vi "Host_9.vi"() -> ()   [LabVIEW 2020]
panel:
  in  "stop":bool
  out "Dane":waveform(dbl)(graph)
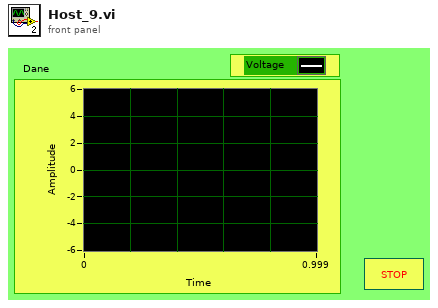
[diagram p1: front panel]
types:
  T1 = enum16{"open", "replace", "create", "open or create", "replace or create", "replace or create with confirmation"}
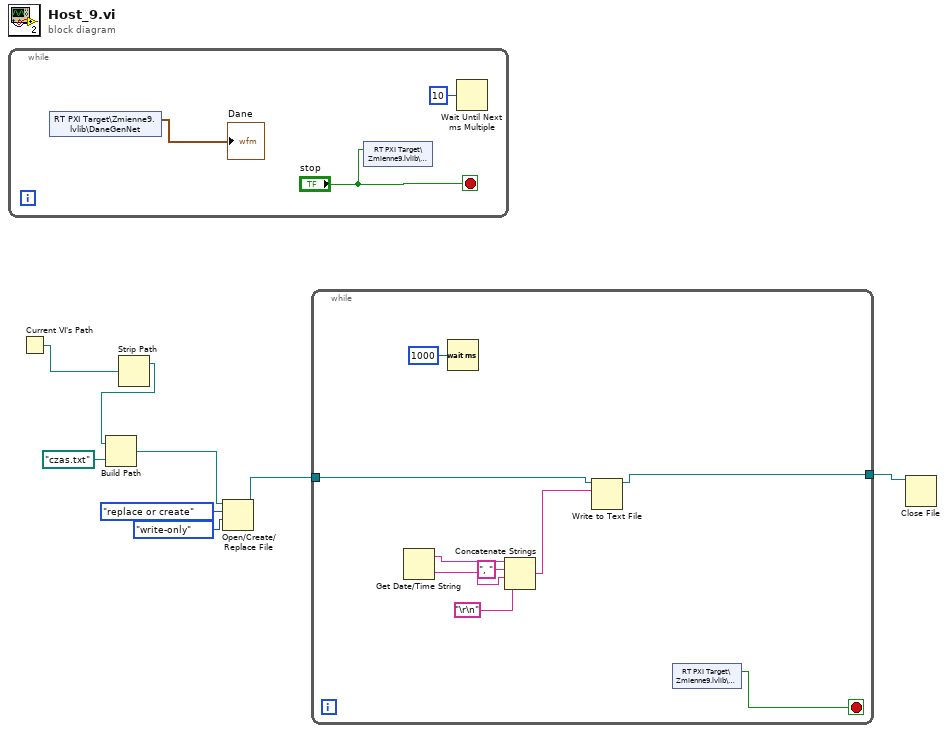
[diagram p0: block diagram]
diagram:
  n1 = while {
    stop <- "stop" stop-if-true
    n2 = shared-variable "RT PXI Target\\Zmienne9.lvlib\\DaneGenNet"() -> (→"Dane":waveform(dbl))  [unwired: 1 in, 1 out]
    n3 = shared-variable "RT PXI Target\\Zmienne9.lvlib\\Stop"("stop") -> ()  [unwired: 1 in, 1 out]
    n4 = Wait Until Next ms Multiple(millisecond multiple=u32 10) -> ()  [unwired: 1 out]
  }
  n5 = Current VI's Path() -> (path=w7:path)
  n6 = Strip Path(path=w7) -> (stripped path=w6:path)  [unwired: 1 out]
  n7 = Build Path(base path=w6, name or relative path=path "czas.txt" ("default name")) -> (appended path=w3:path)
  n8 = Open/Create/Replace File(file path (use dialog)=w3, operation (0:open)=T1."replace or create", access (0:read/write)=enum16{"read/write", "read-only", "write-only"}."write-only") -> (refnum out=w2:refnum<file>)  [unwired: 3 in, 2 out]
  n9 = while {
    tunnel: w2 -> [w13]
    tunnel: [w12] -> w1
    stop <- w15 stop-if-true
    n10 = Get Date/Time String() -> (date string=w19:string, time string=w16:string)  [unwired: 3 in]
    n11 = Wait (ms)(milliseconds to wait=u32 1000) -> ()  [unwired: 1 out]
    n12 = Concatenate Strings(w19, ", " ("string"), w16, "\r\n") -> (w18:string)
    n13 = Write to Text File(file (use dialog)=w13, text=w18) -> (refnum out=w12:refnum<file>)  [unwired: 2 in, 2 out]
    n14 = shared-variable "RT PXI Target\\Zmienne9.lvlib\\Stop"() -> (w15:bool)  [unwired: 1 in, 1 out]
  }
  n15 = Close File(refnum=w1) -> ()  [unwired: 1 in, 2 out]
